vi "sample_main.vi"() -> ()   [LabVIEW 2020]
uses:
  8d1713d4-6516-4828-816a-819b3e449218.vi
panel:
  out "Numeric":dbl
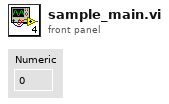
[diagram p1: front panel]
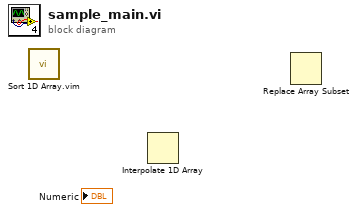
[diagram p0: block diagram]
diagram:
  n1 = call "Sort 1D Array.vim"() -> ()  [unwired: 11 in, 1 out]
  n2 = Interpolate 1D Array() -> ()  [unwired: 2 in, 1 out]
  n3 = Replace Array Subset() -> ()  [unwired: 3 in, 1 out]
